vi "Reset Force.vi"(8 "error in (no error)":errorcluster, 11 "Model in":refnum<class "Model.lvclass">) -> (0 "error out":errorcluster, 3 "Model out":refnum<class "Model.lvclass">)   [LabVIEW 2016, in "Model.lvclass"]
uses:
  Model.lvclass
  Model.lvclass/Model.ctl
  Common_RT_FAILC/FAILC/FAILC.lvclass/FAILC.ctl
  Modbus/DesktopModbus/DesktopModbus.lvclass
  Common_RT_FAILC/FAILC/FAILC.lvclass
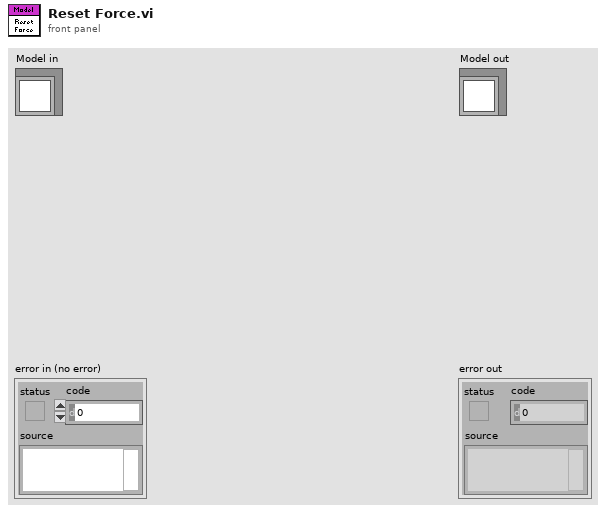
[diagram p1: front panel]
types:
  T1 = typedef "RTFAILC.lvlib/FAData.ctl" = cluster{"Constants":T2, "Command":T3, "Telemetry":T5, "Responses":T6, "Timings":T8}
  T2 = typedef "RTFAILC.lvlib/FAConstants.ctl" = cluster{"ID":i16}
  T3 = typedef "RTFAILC.lvlib/FACommand.ctl" = cluster{"AxialSetPoint":i32, "LateralSetPoint":i32, "PressureServoValveSettings":T4, "BoosterValveSettings":T4}
  T4 = typedef "RTFAILC.lvlib/FAPID.ctl" = cluster{"Kp":sgl, "Ki":sgl, "Kd":sgl, "Kf":sgl}
  T5 = typedef "RTFAILC.lvlib/FATelemetry.ctl" = cluster{"ILCFault":bool, "BroadcastCounter":u8, "AxialLoadCellForce":sgl, "LateralLoadCellForce":sgl, "AxialPressure":T4, "AxialTurbo":T4, "LateralPressure":T4, "LateralTurbo":T4}
  T6 = typedef "RTFAILC.lvlib/FAResponses.ctl" = cluster{"PIDParameters":T7, "ReadPIDParameters":T7, "SetForce":T7, "ForceAndStatus":T7}
  T7 = typedef "RTModbus.lvlib/ExceptionCodes.ctl" = u16
  T8 = typedef "RTFAILC.lvlib/FATimings.ctl" = cluster{"BroadcastSetForce":u32, "PIDParameters":u32, "FreezeSensorValues":u32, "ForceAndStatus":u32, "ReadPIDParameters":u32, "SetForce":u32}
  T9 = typedef "RTModbus.lvlib/TxFrame.ctl" = cluster{"Data":u8[], "WaitForTrigger":bool, "WaitForRx":u16, "TriggerIRQ":bool, "DelayMicroseconds":u16, "DelayMilliseconds":u16, "Timestamp":bool}
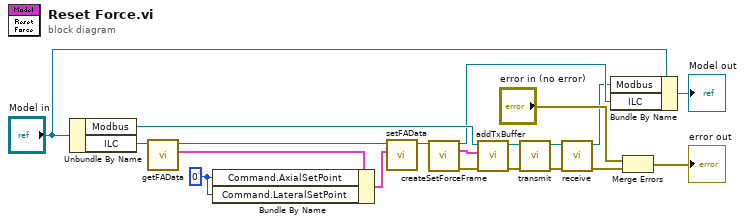
[diagram p0: block diagram]
diagram:
  w16 = 0 ("FACommand.AxialSetPoint")
  n1 = Unbundle By Name("Model in") -> ("Modbus"=w7:refnum<class "DesktopModbus.lvclass">, "ILC"=w6:refnum<class "FAILC.lvclass">)
  n2 = call "getFAData.vi"("FAILC in"=w6) -> ("FAData"=w18:T1, "FAILC out"=w15:refnum<class "FAILC.lvclass">)  [unwired: 9 in]
  n3 = Bundle By Name(cluster=w18, "Command.AxialSetPoint"=w16, "Command.LateralSetPoint"=w16) -> (w17:T1)
  n4 = call "setFAData.vi"("FAData"=w17, "FAILC in"=w15) -> ("FAILC out"=w14:refnum<class "FAILC.lvclass">)  [unwired: 9 in]
  n5 = call-dynamic "createSetForceFrame.vi"("FAILC in"=w14) -> ("FAILC out"=w3:refnum<class "FAILC.lvclass">, "TxFrame"=w13:T9, "error out"=w12:errorcluster)  [unwired: 12 in]
  n6 = call-dynamic "addTxBuffer.vi"("error in (no error)"=w12, "TxFrame"=w13, "DesktopModbus in"=w7) -> ("error out"=w11:errorcluster, "DesktopModbus out"=w8:refnum<class "DesktopModbus.lvclass">)  [unwired: 7 in]
  n7 = call-dynamic "transmit.vi"("error in (no error)"=w11, "DesktopModbus in"=w8) -> ("error out"=w10:errorcluster, "DesktopModbus out"=w9:refnum<class "DesktopModbus.lvclass">)  [unwired: 8 in]
  n8 = call-dynamic "receive.vi"("error in (no error)"=w10, "DesktopModbus in"=w9) -> ("error out"=w1:errorcluster, "DesktopModbus out"=w2:refnum<class "DesktopModbus.lvclass">)  [unwired: 7 in, 1 out]
  n9 = Bundle By Name(cluster="Model in", "Modbus"=w2, "ILC"=w3) -> (→"Model out":refnum<class "Model.lvclass">)
  n10 = Merge Errors("error in (no error)", w1) -> (→"error out":errorcluster)
